vi "initState.vi"(8 "error in (no error)":errorcluster, 9 "Value":dbl, 10 "Num of State":i32=50, 11 "OptCtrl in":refnum<class "OptCtrl.lvclass">) -> (0 "error out":errorcluster, 3 "OptCtrl out":refnum<class "OptCtrl.lvclass">)   [LabVIEW 2016, in "OptCtrl.lvclass"]
doc: "Initialize the state in the basis of degree of freedom."
uses:
  OptCtrl.lvclass
  OptCtrl.lvclass/OptCtrl.ctl
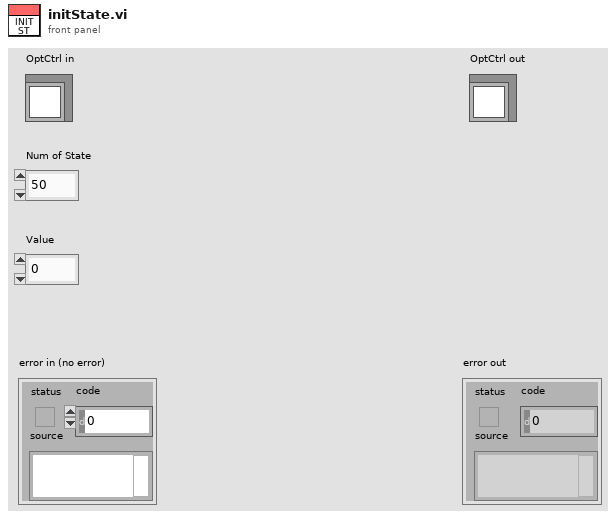
[diagram p1: front panel]
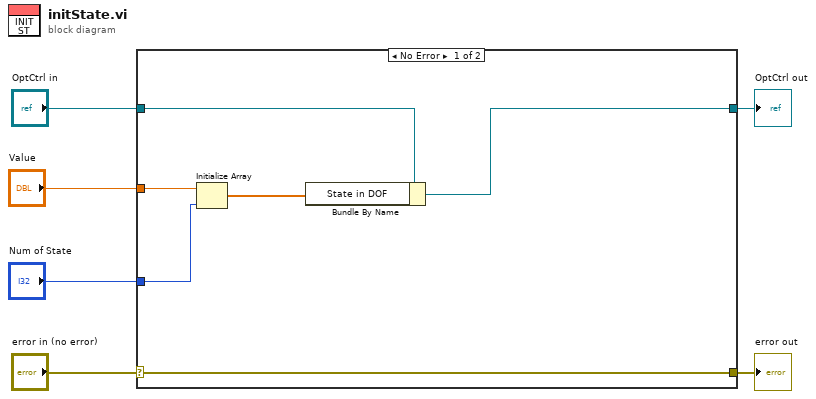
[diagram p0: block diagram]
diagram:
  n1 = case shown="No Error" "error in (no error)" {
    selector: "error in (no error)" -> [w12 w14]
    tunnel: [w12 w14] -> w5
    tunnel: [w7 w13] -> w3
    tunnel: "OptCtrl in" -> [w8 w13]
    tunnel: "Value" -> [w11 _]
    tunnel: "Num of State" -> [w10 _]
    frame No Error {
      n2 = Initialize Array(w11, w10) -> (w9:dbl[])
      n3 = Bundle By Name(cluster=w8, "State in DOF"=w9) -> (w7:refnum<class "OptCtrl.lvclass">)
    }
    frame Error {
    }
  }
  "error out" <- w5
  "OptCtrl out" <- w3
